vi "2283_catapultafinal.vi"(0 "catapulta":bool, 5 "Reset":bool, 9 "cargar en pits":bool, 11 "CAN Talon SRX Ref":T1={"DeviceStatus"={"status"=FALSE, "code"=0, "source"=""}, "Type"=enum."PWM", "PWM"={"PWM Channel"=enum."PWM 1", "DeadBand"={"Name"="", "maxPositivePwm"=0, "minPositivePwm"=0, "centerPwm"=0, "maxNegativePwm"=0, "minNegativePwm"=0, "angularRange"=0}}, "CAN"={"Device Number"=0, "Control Mode"=enum."Percent VBus", "Semaphore"=refnum, "Max Vout"=12.0, "TalonSRX Control Mode"=enum."Percent VBus"}, "Invert"=FALSE}) -> ()   [LabVIEW 2015]
uses:
  <vilib>/Rock Robotics/WPI/MotorControl/WPI_MotorControlDeviceRef.ctl
  <vilib>/Rock Robotics/WPI/MotorControl/WPI_MotorControlType.ctl
  <vilib>/Rock Robotics/SystemInterfaces/DIO/FPGA_DIOPWMChannel.ctl
  <vilib>/Rock Robotics/WPI/PWM/WPI_PWMDeadband.ctl
  <vilib>/Rock Robotics/WPI/CAN/Jaguar/SubVIs/WPI_CANJaguar_ControlMode.ctl
  <vilib>/Rock Robotics/WPI/CAN/TalonSRX/WPI_CANTalonSRX_APIControlMode.ctl
  TypeDefs/estadosCatapulta.ctl
  Globales/Catapulta Disponible Global.vi
  Globales/Feeder Disponible Global.vi
panel:
  out "Catapulta":dbl
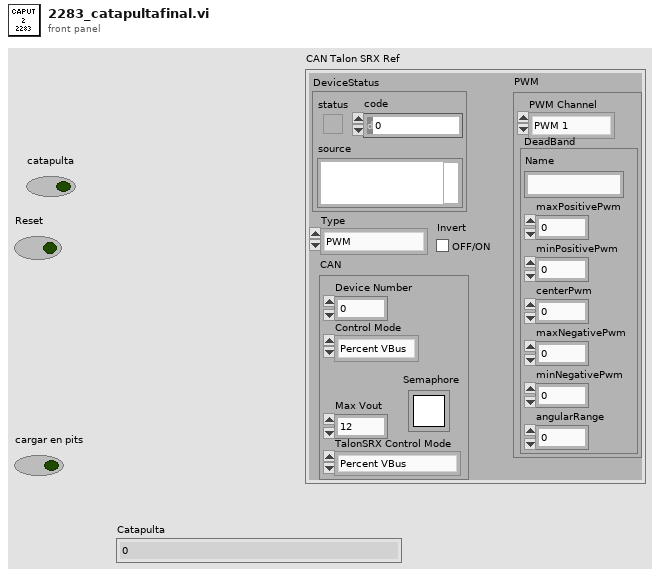
[diagram p1: front panel]
types:
  T1 = typedef "WPI_MotorControlDeviceRef.ctl" = cluster{"DeviceStatus":errorcluster, "Type":T2, "PWM":cluster{"PWM Channel":T3, "DeadBand":T4}, "CAN":cluster{"Device Number":u8, "Control Mode":T5, "Semaphore":T6, "Max Vout":dbl, "TalonSRX Control Mode":T7}, "Invert":bool}
  T2 = typedef "WPI_MotorControlType.ctl" = enum16{"PWM", "CAN", "CANTalonSRX"}
  T3 = typedef "FPGA_DIOPWMChannel.ctl" = enum8{"PWM 0", "PWM 1", "PWM 2", "PWM 3", "PWM 4", "PWM 5", "PWM 6", "PWM 7", "PWM 8", "PWM 9", "PWM MXP 0", "PWM MXP 1", "PWM MXP 2", "PWM MXP 3", "PWM MXP 4", "PWM MXP 5", "PWM MXP 6", "PWM MXP 7", "PWM MXP 8", "PWM MXP 9", "Invalid"}
  T4 = typedef "WPI_PWMDeadband.ctl" = cluster{"Name":string, "maxPositivePwm":i32, "minPositivePwm":i32, "centerPwm":i32, "maxNegativePwm":i32, "minNegativePwm":i32, "angularRange":u16}
  T5 = typedef "WPI_CANJaguar_ControlMode.ctl" = enum8{"Percent VBus", "Current", "Speed", "Position", "Voltage"}
  T6 = typedef "Semaphore RefNum" = refnum<k1>
  T7 = typedef "WPI_CANTalonSRX_APIControlMode.ctl" = enum8{"Percent VBus", "Speed", "Position", "Slave", "Unchanged / Invalid", "Voltage Compensation", "Current", "Motion Profile"}
  T8 = typedef "estadosCatapulta.ctl" = enum16{"timeout", "disparando", "cargado"}
  T9 = typedef "WPI_CANTalonSRX_GlobalStatus.ctl" = cluster{"Applied Throttle":dbl, "Module Enabled":bool, "CAN Error":errorcluster, "Closed Loop Error":dbl, "Forward Limit Switch Closed":bool, "Reverse Limit Switch Closed":bool, "Sensor Position":dbl, "Sensor Velocity":dbl, "Current":dbl, "Sticky Fault - Over Temp":bool, "Sticky Fault - Under Voltage":bool, "Sticky Fault - Forward Limit":bool, "Sticky Fault - Reverse Limit":bool, "Sticky Fault - Forward Soft Limit":bool, "Sticky Fault - Reverse Soft Limit":bool, "Brake is Enabled":bool, "Encoder Position":dbl, "Encoder Velocity":dbl, "Encoder Index Count":dbl, "Encoder A Pin State":bool, "Encoder B Pin State":bool, "Encoder Index Pin State":bool, "Analog In":dbl, "Analog In Velocity":dbl, "Temperature (C)":dbl, "Battery Voltage":dbl, "Control 5 Is Supported":bool, "Current Profile Slot Select":dbl, "Pos Div 8":bool, "Vel Div 4":bool, "Pulse Width Position":i32, "Pulse Width Velocity":i32, "Pulse Width Rise To Rise (us)":i32, "Pulse Width Rise To Fall (us)":i32, "Mot Prof Active Is Under Run":bool, "Mot Prof Active Has Under Run":bool, "Mot Prof Active Is Last":bool, "Mot Prof Active Velocity Only":bool, "Mot Prof Active Is Valid":bool, "Mot Prof Buffer Is Full":bool, "Mot Prof Active Profile Slot Select":i32, "Mot Prof NextID":i32, "Mot Prof Count":i32, "Mot Prof Active Velocity":dbl, "Mot Prof Active Position":dbl, "Mot Prof Output Enable":i32}
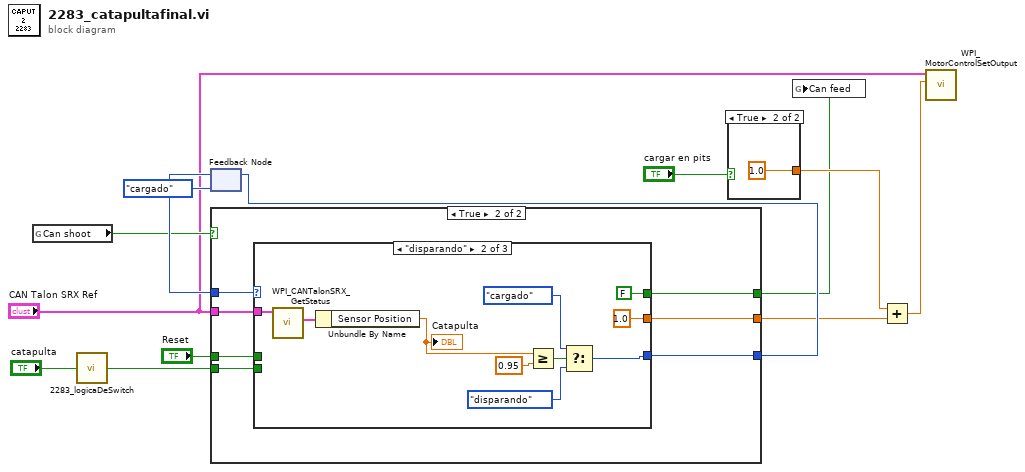
[diagram p0: block diagram]
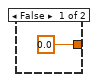
[diagram p2: hidden frame]
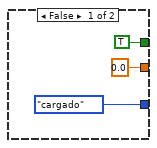
[diagram p3: hidden frame]
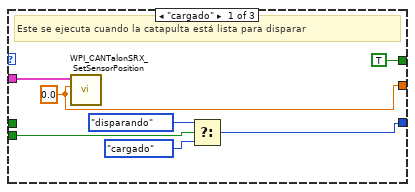
[diagram p4: hidden frame]
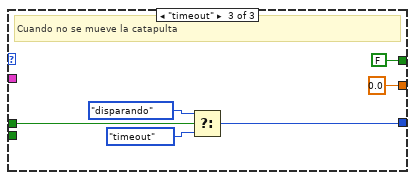
[diagram p5: hidden frame]
diagram:
  n1 = global read "Catapulta Disponible Global.vi" "Can shoot"() -> (w6:bool)
  n2 = call "2283_logicaDeSwitch.vi"("Input"="catapulta") -> ("Output"=w4:bool)
  n3 = feedback #1(estadosCatapulta."cargado") -> (w12:T8)
  n4 = case shown="True" w6 {
    tunnel: w12 -> [_ w23]
    tunnel: [estadosCatapulta."cargado" w22] -> w11
    tunnel: w4 -> [_ w21]
    tunnel: "Reset" -> [_ w20]
    tunnel: [0.0 w19] -> w9
    tunnel: [TRUE w18] -> w7
    tunnel: "CAN Talon SRX Ref" -> [_ w17]
    frame False {
    }
    frame True {
      n5 = case shown="\"disparando\"" w23 {
        tunnel: [w29 w38 w44] -> w22
        tunnel: w21 -> [w30 _ _]
        tunnel: w20 -> [_ _ w46]
        tunnel: [w24 1.0 0.0] -> w19
        tunnel: [TRUE FALSE FALSE] -> w18
        tunnel: w17 -> [w25 w31 _]
        frame "cargado" {
          w24 = 0.0 ("Numeric")
          # "Este se ejecuta cuando la catapulta está lista para disparar"
          n6 = call <vilib>:"WPI_CANTalonSRX_SetSensorPosition.vi"("New Sensor Position"=w24, "CAN Talon SRX Ref"=w25) -> ()  [unwired: 8 in, 2 out]
          n7 = Select(t=estadosCatapulta."disparando", s=w30, f=estadosCatapulta."cargado") -> (s? t:f=w29:T8)
        }
        frame "disparando" {
          n8 = call <vilib>:"WPI_CANTalonSRX_GetStatus.vi"("CAN Talon SRX Ref"=w31) -> ("Talon SRX Status"=w36:T9)  [unwired: 8 in, 2 out]
          n9 = Unbundle By Name(w36) -> ("Sensor Position"=w34:dbl)
          "Catapulta" <- w34
          n10 = Greater Or Equal?(x=w34, y=0.95) -> (x >= y?=w32:bool)
          n11 = Select(t=estadosCatapulta."cargado", s=w32, f=estadosCatapulta."disparando") -> (s? t:f=w38:T8)
        }
        frame "timeout" {
          # "Cuando no se mueve la catapulta"
          n12 = Select(t=estadosCatapulta."disparando", s=w46, f=estadosCatapulta."timeout") -> (s? t:f=w44:T8)
        }
      }
    }
  }
  n13 = feedback-in #1(w11) -> ()
  n14 = case shown="True" "cargar en pits" {
    tunnel: [0.0 ("Numeric") 1.0] -> w8
    frame False {
    }
    frame True {
    }
  }
  n15 = global write "Feeder Disponible Global.vi" "Can feed"(w7) -> ()
  n16 = Add(x=w8, y=w9) -> (x+y=w3:dbl)
  n17 = call <vilib>:"WPI_MotorControlSetOutput.vi"("Output"=w3, "MotorControlDevRef"="CAN Talon SRX Ref") -> ()  [unwired: 7 in, 3 out]
